vi "Initialize_DSC.vi"   [LabVIEW 2016]
uses:
  <vilib>/addons/_JKI.lib/Serialization/JSON/JKI JSON Serialization.lvlib
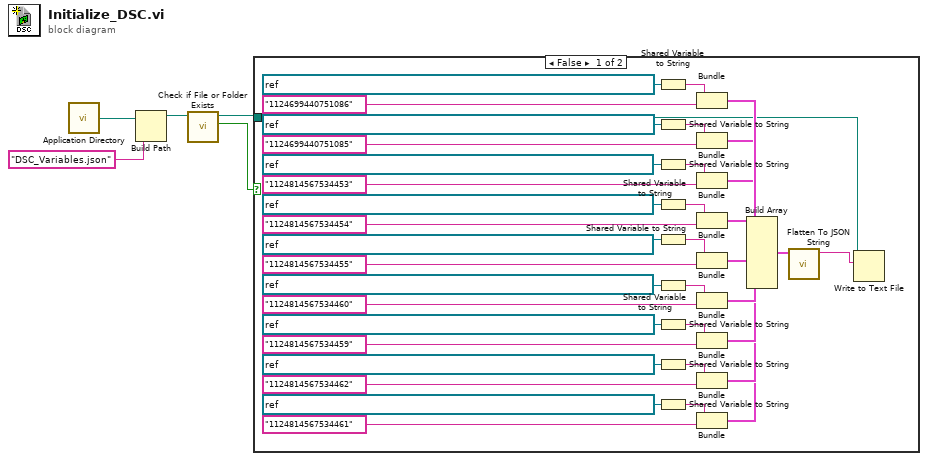
[diagram p0: block diagram]
diagram:
  n1 = call <vilib>:"Application Directory.vi"() -> ("Application Directory"=w1:path)
  n2 = Build Path(base path=w1, name or relative path="DSC_Variables.json") -> (appended path=w4:path)
  n3 = call <vilib>:"Check if File or Folder Exists.vi"("path"=w4) -> ("file or folder exists?"=w2:bool, "dup path"=w3:path)  [unwired: 8 in, 1 out]
  n4 = case shown="False" w2 {
    tunnel: w3 -> [w6 _]
    frame False {
      n5 = Shared Variable to String(1:refnum<k21> "ni.var.psp://housesoftheholy/PPMS 1/PPMS 1 Magnetic Field" ("shared variable refnum in")) -> (0:w18:string)
      n6 = Shared Variable to String(1:refnum<k21> "ni.var.psp://housesoftheholy/PPMS 1/PPMS 1 Temperature" ("shared variable refnum in")) -> (0:w20:string)
      n7 = Shared Variable to String(1:refnum<k21> "ni.var.psp://housesoftheholy/PPMS 2/PPMS 2 Temperature" ("shared variable refnum in 3")) -> (0:w22:string)
      n8 = Shared Variable to String(1:refnum<k21> "ni.var.psp://housesoftheholy/PPMS 2/PPMS 2 Magnetic Field" ("shared variable refnum in 4")) -> (0:w24:string)
      n9 = Shared Variable to String(1:refnum<k21> "ni.var.psp://housesoftheholy/PPMS 2/PPMS 2 Helium Level" ("shared variable refnum in 5")) -> (0:w26:string)
      n10 = Shared Variable to String(1:refnum<k21> "ni.var.psp://housesoftheholy/Montana THZ 1/THZ 1 Temperature" ("shared variable refnum in 6")) -> (0:w28:string)
      n11 = Shared Variable to String(1:refnum<k21> "ni.var.psp://housesoftheholy/Cypher/Cypher Temperature" ("shared variable refnum in 9")) -> (0:w30:string)
      n12 = Shared Variable to String(1:refnum<k21> "ni.var.psp://housesoftheholy/MNK_18T/MNK_TC_T3" ("shared variable refnum in 10")) -> (0:w32:string)
      n13 = Shared Variable to String(1:refnum<k21> "ni.var.psp://housesoftheholy/MFP3D/MFP3D Temperature" ("shared variable refnum in 11")) -> (0:w34:string)
      n14 = Bundle(w18, "1124699440751086") -> (w17:cluster{string, string})  [unwired: 1 in]
      n15 = Bundle(w20, "1124699440751085") -> (w16:cluster{string, string})  [unwired: 1 in]
      n16 = Bundle(w22, "1124814567534453") -> (w15:cluster{string, string})  [unwired: 1 in]
      n17 = Bundle(w24, "1124814567534454") -> (w14:cluster{string, string})  [unwired: 1 in]
      n18 = Bundle(w26, "1124814567534455") -> (w13:cluster{string, string})  [unwired: 1 in]
      n19 = Bundle(w28, "1124814567534460") -> (w12:cluster{string, string})  [unwired: 1 in]
      n20 = Bundle(w30, "1124814567534459") -> (w11:cluster{string, string})  [unwired: 1 in]
      n21 = Bundle(w32, "1124814567534462") -> (w10:cluster{string, string})  [unwired: 1 in]
      n22 = Bundle(w34, "1124814567534461") -> (w9:cluster{string, string})  [unwired: 1 in]
      n23 = Build Array(w17, w16, w15, w14, w13, w12, w11, w10, w9) -> (w8:cluster{string, string}[])
      n24 = call <vilib>:"Flatten To JSON String.vi"("Variant"=w8) -> ("JSON String"=w7:string)  [unwired: 9 in, 1 out]
      n25 = Write to Text File(file (use dialog)=w6, text=w7) -> ()  [unwired: 2 in, 3 out]
    }
    frame True {
    }
  }
